vi "TPNT_StartAsyncDDSServer.vi"(4 "notifier":refnum<notifier>, 5 "updaterate":refnum<vi>, 6 "stop":refnum<vi>, 7 "async":refnum<vi>, 8 "error in (no error)":errorcluster, 9 "stream_name":string, 10 "utc":refnum<vi>) -> (0 "error out":errorcluster)   [LabVIEW 2016]
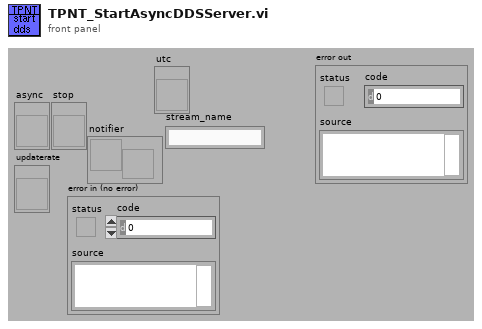
[diagram p1: front panel]
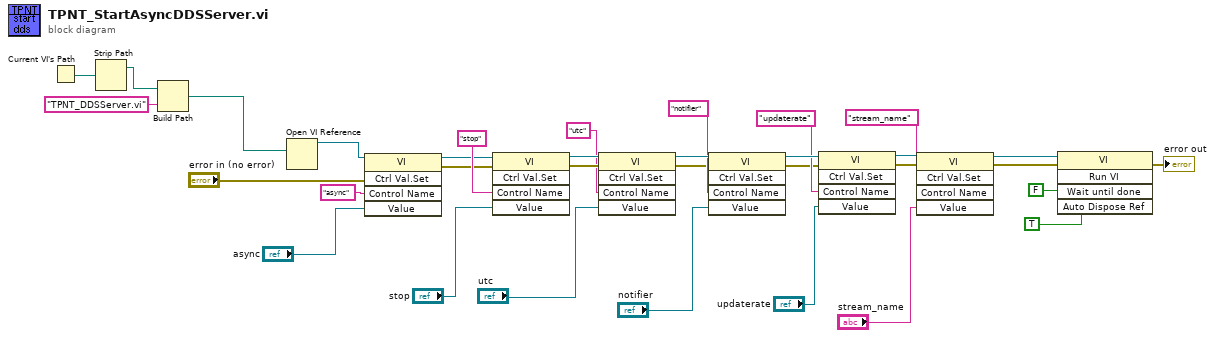
[diagram p0: block diagram]
diagram:
  n1 = Current VI's Path() -> (path=w16:path)
  n2 = Strip Path(path=w16) -> (stripped path=w15:path)  [unwired: 1 out]
  n3 = Build Path(base path=w15, name or relative path="TPNT_DDSServer.vi") -> (appended path=w13:path)
  n4 = Open VI Reference(vi path=w13) -> (vi reference=w33:refnum<vi>)  [unwired: 1 in, 5 out]
  n5 = invoke class="VI" method="Ctrl Val.Set"(reference=w33, error in="error in (no error)", "Control Name"="async", "Value"="async") -> (reference out=w30:refnum<vi>, error out=w10:errorcluster)  [unwired: 1 in, 3 out]
  n6 = invoke class="VI" method="Ctrl Val.Set"(reference=w30, error in=w10, "Control Name"="stop", "Value"="stop") -> (reference out=w29:refnum<vi>, error out=w28:errorcluster)  [unwired: 1 in, 3 out]
  n7 = invoke class="VI" method="Ctrl Val.Set"(reference=w29, error in=w28, "Control Name"="utc", "Value"="utc") -> (reference out=w26:refnum<vi>, error out=w9:errorcluster)  [unwired: 1 in, 3 out]
  n8 = invoke class="VI" method="Ctrl Val.Set"(reference=w26, error in=w9, "Control Name"="notifier", "Value"="notifier") -> (reference out=w23:refnum<vi>, error out=w8:errorcluster)  [unwired: 1 in, 3 out]
  n9 = invoke class="VI" method="Ctrl Val.Set"(reference=w23, error in=w8, "Control Name"="updaterate", "Value"="updaterate") -> (reference out=w6:refnum<vi>, error out=w5:errorcluster)  [unwired: 1 in, 3 out]
  n10 = invoke class="VI" method="Ctrl Val.Set"(reference=w6, error in=w5, "Control Name"="stream_name", "Value"="stream_name") -> (reference out=w4:refnum<vi>, error out=w3:errorcluster)  [unwired: 1 in, 3 out]
  n11 = invoke class="VI" method="Run VI"(reference=w4, error in=w3, "Wait until done"=FALSE ("Wait Until Done"), "Auto Dispose Ref"=TRUE ("Auto Dispose Reference")) -> (error out=→"error out":errorcluster)  [unwired: 1 in, 4 out]
